vi "GEvt-Generate State Change Log.vi"(0 "CSM Global Log Event":T4, 1 "Current State":string, 2 "Arguments":string, 3 "Source Message.*State":string, 4 "Source Message.*Arguments":string, 5 "Source Module":string, 6 "Name (\"\" to Use UUID)":string, 10 "CSM:LogFilter.lvclass":refnum<class "LogFilter.lvclass">) -> (14 "CSM Global Log Event Out":T4, 16 "Event Data":T1={"Name (\"\" to Use UUID)"="", "Current State"="", "Arguments"="", "Source Message"={"‘State"="", "’Arguments"="", "’Error"={"status"=FALSE, "code"=0, "source"=""}}, "Source Module"="", "Complete(T)/Start(F)"=FALSE, "LogType"=enum."State Change", "Time Stamp"=timestamp(0 s since 1904-01-01)})   [LabVIEW 2017, in "Communicable State Machine.lvlib"]
doc: "### GEvt-Generate State Change Log.vi\n\n-- <b>Controls</b> --\n- <b>CSM Global Log Event</b>:\n- <b>Current State</b>:\n- <b>Arguments</b>:\n- <b>Source Message.*State</b>:\n- <b>Source Message.*Arguments</b>:\n- <b>Source Module</b>:\n- <b>Name(\"\" to use uuid)</b>:\n- <b>CSM:LogFilter.lvclass</b>:\n\n-- <b>Indicators</b> --\n- <b>CSM Global Log Event out</b>:\n- <b>event data</b>:"
uses:
  Communicable State Machine.lvlib
  GEvt-Refs.ctl
  Typedef/_CSM_GlobalLog_MSG.ctl
  Typedef/_CSM_Response Source Message.ctl
  Typedef/_CSM_GlobalLog_MSG_TYPE.ctl
  LogFilter/LogFilter.lvclass
  LogFilter/LogFilter - Check.vi
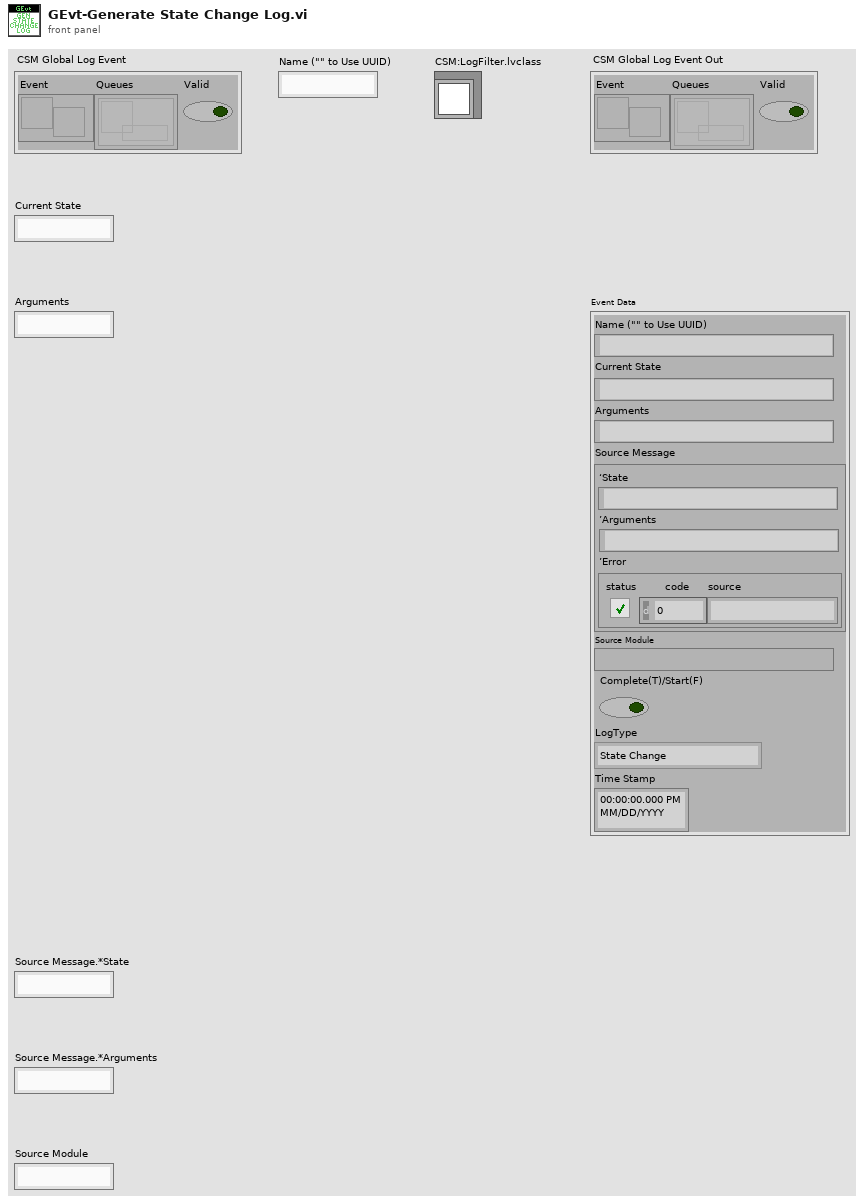
[diagram p1: front panel]
types:
  T1 = typedef "Communicable State Machine.lvlib/_CSM_GlobalLog_MSG.ctl" = cluster{"Name (\"\" to Use UUID)":string, "Current State":string, "Arguments":string, "Source Message":T2, "Source Module":string, "Complete(T)/Start(F)":bool, "LogType":T3, "Time Stamp":timestamp}
  T2 = typedef "Communicable State Machine.lvlib/_CSM_Response Source Message.ctl" = cluster{"‘State":string, "’Arguments":string, "’Error":errorcluster}
  T3 = typedef "Communicable State Machine.lvlib/_CSM_GlobalLog_MSG_TYPE.ctl" = enum16{"User Log", "State Change", "Status", "Interrupt", "Register", "Unregister", "Error Log", "Module Created", "Module Destroyed"}
  T4 = typedef "Communicable State Machine.lvlib/GEvt-Refs.ctl" = cluster{"Event":refnum<user-event>, "Queues":refnum<queue>[], "Valid":bool}
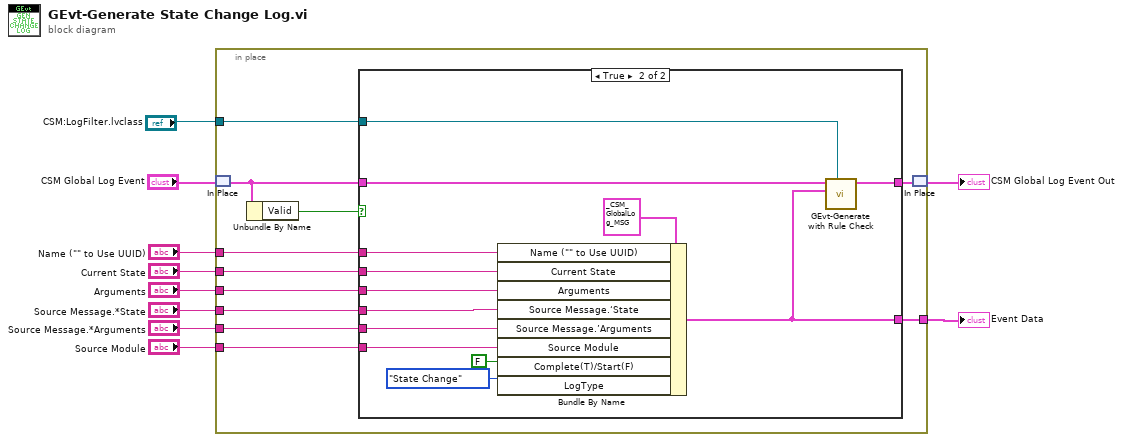
[diagram p0: block diagram]
diagram:
  n1 = in-place {
    in-place-border: [w20] -> w8
    in-place-border: "Name (\"\" to Use UUID)" -> [w19]
    in-place-border: "Current State" -> [w18]
    in-place-border: "Arguments" -> [w17]
    in-place-border: "Source Message.*State" -> [w16]
    in-place-border: "Source Message.*Arguments" -> [w15]
    in-place-border: "Source Module" -> [w14]
    in-place-border: "CSM:LogFilter.lvclass" -> [w13]
    n2 = in-place-match #1("CSM Global Log Event") -> (w12:T4)
    n3 = Unbundle By Name(w12) -> ("Valid"=w11:bool)
    n4 = case shown="True" w11 {
      tunnel: w12 -> [w22 w35]
      tunnel: [w22 w34] -> w21
      tunnel: [_ w23] -> w20
      tunnel: w19 -> [_ w30]
      tunnel: w18 -> [_ w29]
      tunnel: w17 -> [_ w28]
      tunnel: w16 -> [_ w27]
      tunnel: w15 -> [_ w26]
      tunnel: w14 -> [_ w25]
      tunnel: w13 -> [_ w24]
      frame False {
      }
      frame True {
        n5 = Bundle By Name(cluster=T1 {"Name (\"\" to Use UUID)"="", "Current State"="", "Arguments"="", "Source Message"={"‘State"="", "’Arguments"="", "’Error"={"status"=FALSE, "code"=0, "source"=""}}, "Source Module"="", "Complete(T)/Start(F)"=FALSE, "LogType"=enum."State Change", "Time Stamp"=timestamp(0 s since 1904-01-01)} ("event data"), "Name (\"\" to Use UUID)"=w30, "Current State"=w29, "Arguments"=w28, "Source Message.‘State"=w27, "Source Message.’Arguments"=w26, "Source Module"=w25, "Complete(T)/Start(F)"=FALSE, "LogType"=_CSM_GlobalLog_MSG_TYPE."State Change" ("Type")) -> (w23:T1)
        n6 = call "GEvt-Generate with Rule Check.vi"("LogFilter In"=w24, "Event Data"=w23, "CSM Global Log Event In"=w35) -> ("CSM Global Log Event Out"=w34:T4)  [unwired: 8 in]
      }
    }
    n7 = in-place-match #1(w21) -> (→"CSM Global Log Event Out":T4)
  }
  "Event Data" <- w8
